vi "ma_Check Tone (CDB).vi"(10 "fs":dbl, 11 "tone info":T2 {"phase [degree]" format="%.2f"; "amplitude" format="%.2f"; "frequency" format="%.5f"}) -> (3 "measurement info":T1={"uncertainty"=0.0, "Warning"=FALSE, "comments"="reserved for future use"} {"uncertainty" format="%0.2p"})   [LabVIEW 2020, in "NI_MAPro.lvlib"]
uses:
  NI_MAPro.lvlib
panel:
  in  "error 3":string="Failed to detect tone phase"
  in  "error 2":string="Failed to detect tone frequency"
  in  "error":string="Failed to detect tone amplitude"
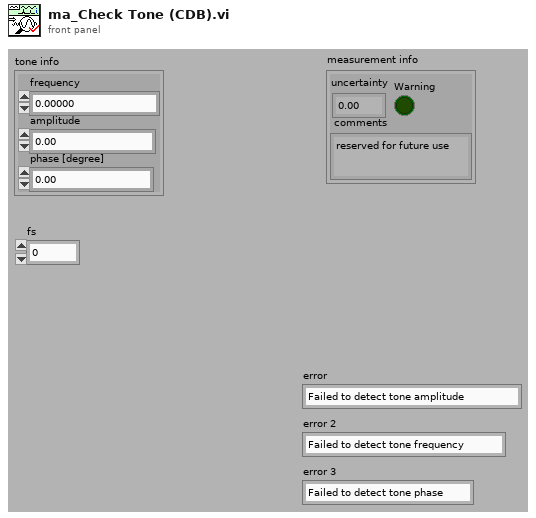
[diagram p1: front panel]
types:
  T1 = cluster{"uncertainty":dbl, "Warning":bool, "comments":string}
  T2 = cluster{"frequency":dbl, "amplitude":dbl, "phase [degree]":dbl}
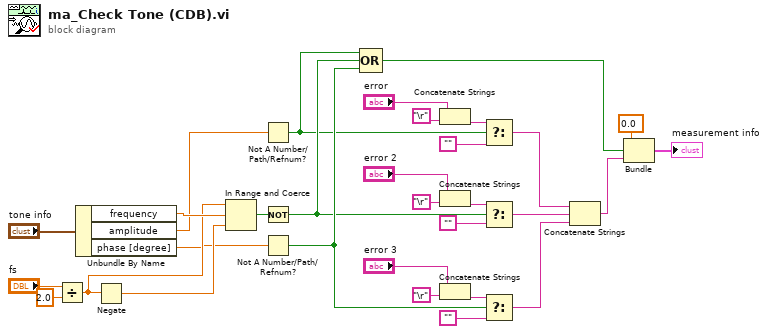
[diagram p0: block diagram]
diagram:
  n1 = Divide(x="fs", y=2.0) -> (x/y=w25:dbl)
  n2 = Unbundle By Name("tone info") -> ("frequency"=w29:dbl, "amplitude"=w22:dbl, "phase [degree]"=w14:dbl)
  n3 = Negate(x=w25) -> (-x=w26:dbl)
  n4 = In Range and Coerce(upper limit=w25, x=w29, lower limit=w26) -> (In Range?=w30:bool)  [unwired: 1 out]
  n5 = Not A Number/Path/Refnum?(number/path/refnum=w22) -> (NaN/Path/Refnum?=w8:bool)
  n6 = Not(x=w30) -> (.not. x?=w9:bool)
  n7 = Not A Number/Path/Refnum?(number/path/refnum=w14) -> (NaN/Path/Refnum?=w10:bool)
  n8 = Compound Arithmetic op=OR(w8, w9, w10) -> (w6:bool)
  n9 = Concatenate Strings("error", "\r") -> (w21:string)
  n10 = Concatenate Strings("error 2", "\r") -> (w23:string)
  n11 = Concatenate Strings("error 3", "\r") -> (w16:string)
  n12 = Select(t=w21, s=w8, f="") -> (s? t:f=w5:string)
  n13 = Select(t=w23, s=w9, f="") -> (s? t:f=w4:string)
  n14 = Select(t=w16, s=w10, f="") -> (s? t:f=w3:string)
  n15 = Concatenate Strings(w5, w4, w3) -> (w2:string)
  n16 = Bundle(0.0, w6, w2) -> (→"measurement info":cluster{dbl, bool, string})  [unwired: 1 out]
